vi "display_stats.vi"(8 "error in":errorcluster, 9 "Variables":T1, 10 "catch stats":refnum<vi>, 11 "stim stats":refnum<vi>) -> (0 "error out":errorcluster)   [LabVIEW 2016]
uses:
  Type Definitions/vars_runtime.ctl
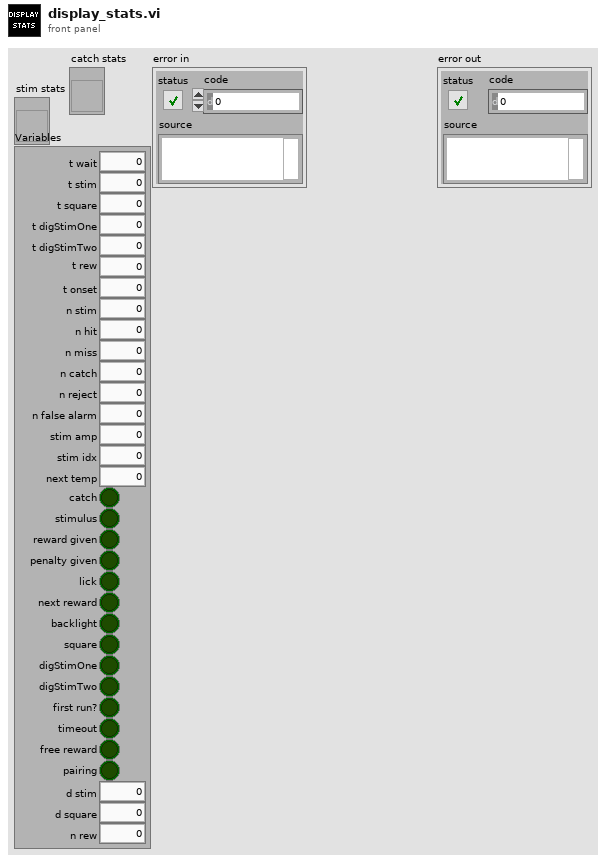
[diagram p1: front panel]
types:
  T1 = typedef "vars_runtime.ctl" = cluster{"t wait":u16, "t stim":u16, "t square":u16, "t digStimOne":u16, "t digStimTwo":u16, "t rew":u16, "t onset":u32, "n stim":u16, "n hit":u16, "n miss":u16, "n catch":u16, "n reject":u16, "n false alarm":u16, "stim amp":sgl, "stim idx":i32, "next temp":sgl, "catch":bool, "stimulus":bool, "reward given":bool, "penalty given":bool, "lick":bool, "next reward":bool, "backlight":bool, "square":bool, "digStimOne":bool, "digStimTwo":bool, "first run?":bool, "timeout":bool, "free reward":bool, "pairing":bool, "d stim":u16, "d square":u16, "n rew":u16}
  T2 = cluster{"n catch":u16, u16, "n false alarm":u16, dbl}
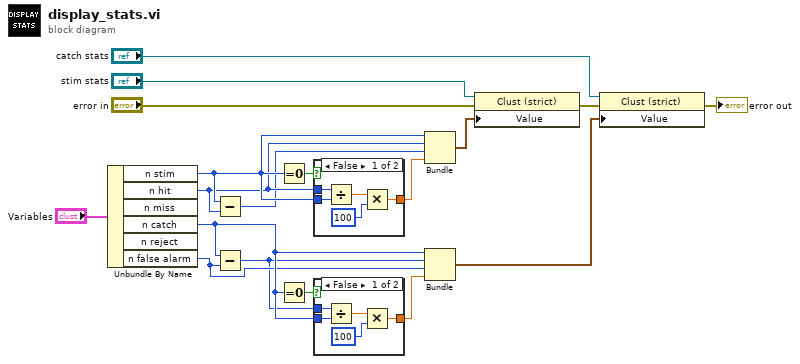
[diagram p0: block diagram]
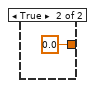
[diagram p2: hidden frame]
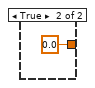
[diagram p3: hidden frame]
diagram:
  n1 = Unbundle By Name("Variables") -> ("n stim"=w6:u16, "n hit"=w5:u16, "n catch"=w3:u16, "n false alarm"=w2:u16)  [unwired: 2 out]
  n2 = Subtract(x=w6, y=w5) -> (x-y=w4:u16)
  n3 = Subtract(x=w3, y=w2) -> (x-y=w1:u16)
  n4 = Equal To 0?(x=w6) -> (x = 0?=w15:bool)
  n5 = Equal To 0?(x=w3) -> (x = 0?=w12:bool)
  n6 = case shown="False" w15 {
    tunnel: w5 -> [w23 _]
    tunnel: w6 -> [w20 _]
    tunnel: [w19 0.0] -> w14
    frame False {
      n7 = Divide(x=w23, y=w20) -> (x/y=w22:dbl)
      n8 = Multiply(x=w22, y=100) -> (x*y=w19:dbl)
    }
    frame True {
    }
  }
  n9 = case shown="False" w12 {
    tunnel: w1 -> [w29 _]
    tunnel: w3 -> [w26 _]
    tunnel: [w25 0.0] -> w13
    frame False {
      n10 = Divide(x=w29, y=w26) -> (x/y=w28:dbl)
      n11 = Multiply(x=w28, y=100) -> (x*y=w25:dbl)
    }
    frame True {
    }
  }
  n12 = Bundle("n stim"=w6, "n hit"=w5, w4, w14) -> (w18:cluster{"n stim":u16, "n hit":u16, u16, dbl})  [unwired: 1 in]
  n13 = Bundle("n catch"=w3, w1, "n false alarm"=w2, w13) -> (w9:T2)  [unwired: 1 in]
  n14 = property class="Clust (strict)"(reference="stim stats", error in="error in", "Value"=w18) -> (error out=w10:errorcluster)  [unwired: 1 out]
  n15 = property class="Clust (strict)"(reference="catch stats", error in=w10, "Value"=w9) -> (error out=→"error out":errorcluster)  [unwired: 1 out]
